vi "HTSuperProWriteAnalog.vi"(1 "Port":T2 items=["Port 1", "Port 2", "Port 3", "Port 4"], 2 "NXT":T1={"error"={"status"=FALSE, "code"=0, "source"=""}, "address"="", "NXT #"=-1, "Show Error"=TRUE, "Connection"=4} {"Connection" items=["USB", "Bluetooth", "USB then Bluetooth", "Last Connection", "Preference"]}, 3 "Voltage":i16=1023 min=0 max=1023 step=1, 4 "Frequency":i16=1 min=1 max=8191 step=1, 5 "Analog Mode":u8(ring) items=["DC", "Sine Wave", "Square Wave", "Pos Sawtooth Wave", "Neg Sawtooth Wave", "Triangle Wave", "PWM Voltage"], 6 "Analog Output":u8(ring) items=["O0", "O1"]) -> (0 "NXT":T1={"error"={"status"=FALSE, "code"=0, "source"=""}, "address"="", "NXT #"=-1, "Show Error"=TRUE, "Connection"=4} {"Connection" items=["USB", "Bluetooth", "USB then Bluetooth", "Last Connection", "Preference"]})   [LabVIEW 2009]
doc: "HiTechnic SuperPro - Write Analog Port\n\n<B>Inputs\nPort </B> is the port connected to the sensor. Port 1 is the default, but Port 2, Port 3, or Port 4 can also be selected.\n<B>NXT </B> connects to NXT terminal of previous VI to establish the flow of the program.\n<B>Analog Output </B> specify either O0 or O1 output port.\n<B>Analog Mode</B> specify one of 7 analog modes: DC, Sine wave, Square wave, Positive sawtooth wave, Negative sawtooth wave, Triangle wave, or PWM.\n<B>Frequency </B> specify the frequency, in Hertz, used for one of analog wave form. Range is 1 to 8191Hz (vibrations per second).\n<B>Voltage </B> specify the voltage level of the analog output. Range is 0 to 1023 which corresponds to 0 to 3.3v. Note that for Sine, Square, Sawtooth, and Triangle waves, the output signal is centered at 1.65 v and the specified voltage is the range from min to max. \n\n<B>Outputs\nNXT </B> wires to NXT terminal of next VI to establish the flow of the program."
uses:
  <vilib>/NXT/Block Support/NXT_InputPort.ctl
  <vilib>/NXT/Subs/LVHSConnector.ctl
  <vilib>/NXT/Block Support/HWPage.SensorType.ctl
  <vilib>/NXT/Block Support/HWPage.SensorMode.ctl
panel:
  # "Analog Output:\nO0, O1"
  # "Analog Mode:\nDC, Sine, Square, PosSawtooth, NegSawtooth, Triangle, or PWM"
  # "Frequency range:\n1 - 8191"
  # "Voltage Value 0-1023\ncorresponds to 0-3.3v"
  # "HiTechnic SuperPro Prototype board VI\nWrite Analog Port\n\nSet the output paramters to one of the two analog output ports on the SuperPro.\n\n(c) HiTechnic 2011"
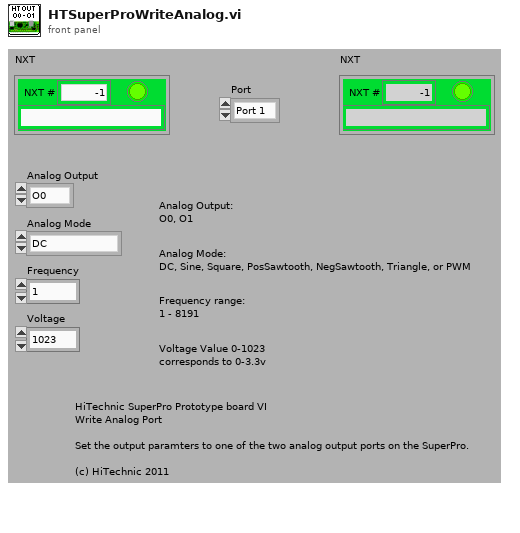
[diagram p1: front panel]
types:
  T1 = typedef "LVHSConnector.ctl" = cluster{"error":errorcluster, "address":string, "NXT #":i32, "Show Error":bool, "Connection":u16}
  T2 = typedef "NXT_InputPort.ctl" = u8
  T3 = typedef "HWPage.SensorType.ctl" = u8
  T4 = typedef "HWPage.SensorMode.ctl" = u8
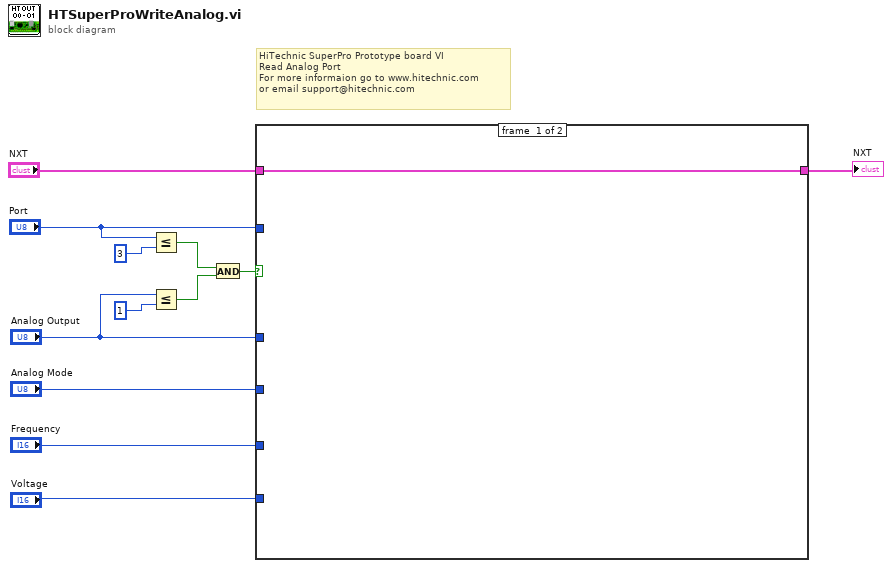
[diagram p0: block diagram]
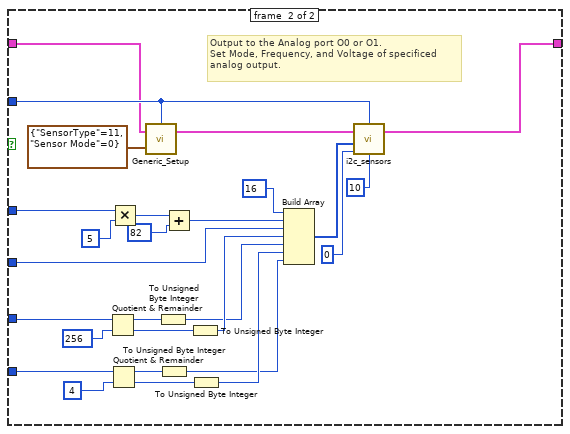
[diagram p2: hidden frame]
diagram:
  # "HiTechnic SuperPro Prototype board VI\nRead Analog Port\nFor more informaion go to www.hitechnic.com\nor email support@hitechnic.com"
  n1 = Less Or Equal?(x="Port", y=u8 3) -> (x <= y?=w7:bool)
  n2 = Less Or Equal?(x="Analog Output", y=u8 1) -> (x <= y?=w8:bool)
  n3 = And(x=w7, y=w8) -> (x .and. y?=w6:bool)
  n4 = case shown="True" w6 {
    tunnel: "Port" -> [_ w38]
    tunnel: "Analog Output" -> [_ w40]
    tunnel: "NXT" -> [w13 w37]
    tunnel: [w13 w35] -> w10
    tunnel: "Analog Mode" -> [_ w27]
    tunnel: "Frequency" -> [_ w26]
    tunnel: "Voltage" -> [_ w17]
    frame #0 {
    }
    frame #1 {
      # "Output to the Analog port O0 or O1.\nSet Mode, Frequency, and Voltage of specificed\nanalog output."
      n5 = Quotient & Remainder(x=w26, y=i16 256) -> (x-y*floor(x/y)=w24:i16, floor(x/y)=w23:i16)
      n6 = Quotient & Remainder(x=w17, y=i16 4) -> (x-y*floor(x/y)=w19:i16, floor(x/y)=w20:i16)
      n7 = Multiply(x=w40, y=u8 5) -> (x*y=w33:u8)
      n8 = call <vilib>:"Generic_Setup.vi"("Sensor Setup"=cluster{"SensorType":T3, "Sensor Mode":T4} {"SensorType"=11, "Sensor Mode"=0}, "NXT"=w37, "Port"=w38) -> ("NXT"=w36:T1)  [unwired: 1 out]
      n9 = To Unsigned Byte Integer(number=w24) -> (unsigned 8bit integer=w21:u8)
      n10 = To Unsigned Byte Integer(number=w19) -> (unsigned 8bit integer=w15:u8)
      n11 = Add(x=w33, y=u8 82) -> (x+y=w30:u8)
      n12 = To Unsigned Byte Integer(number=w23) -> (unsigned 8bit integer=w22:u8)
      n13 = To Unsigned Byte Integer(number=w20) -> (unsigned 8bit integer=w16:u8)
      n14 = Build Array(u8 16, w30, w27, w22, w21, w16, w15) -> (w29:u8[])
      n15 = call <vilib>:"i2c_sensors.vi"("Return Length"=u8 0, "Bytes to Write"=w29, "Wait (msec)"=u32 10, "NXT"=w36, "Port"=w38) -> ("NXT"=w35:T1)  [unwired: 2 out]
    }
  }
  "NXT" <- w10
